vi "遥控器IP地址参数.vi"(10 "数组":u8[](array[numeric]), 11 "ID_VCU_MCU_1输入":u32=150013185 format="0x%x") -> (3 "Send":T1)   [LabVIEW 2016]
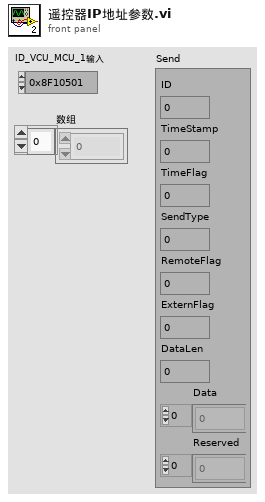
[diagram p1: front panel]
types:
  T1 = typedef "ControlCAN.lvlib/VCI_CAN_OBJ.ctl" = cluster{"ID":u32, "TimeStamp":u32, "TimeFlag":u8, "SendType":u8, "RemoteFlag":u8, "ExternFlag":u8, "DataLen":u8, "Data":u8[], "Reserved":u8[]}
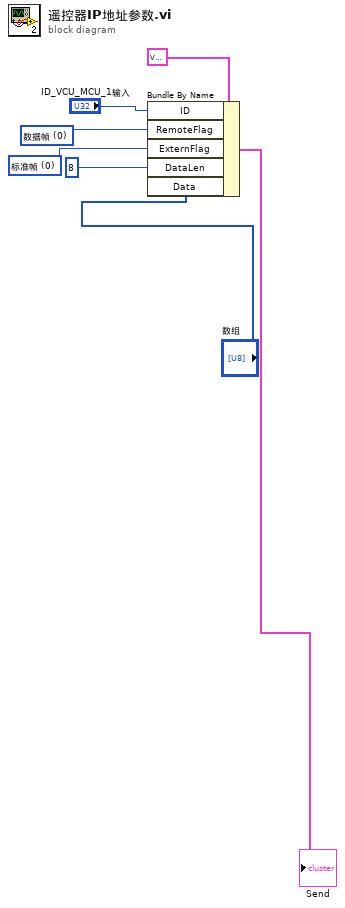
[diagram p0: block diagram]
diagram:
  w4 = u8 0 items=["标准帧", "扩展帧"] ("Format 2")
  w5 = u8 0 items=["数据帧", "远程帧"] ("Type 2")
  n1 = Bundle By Name(cluster=T1 {"ID"=0, "TimeStamp"=0, "TimeFlag"=0, "SendType"=0, "RemoteFlag"=0, "ExternFlag"=0, "DataLen"=0, "Data"=[], "Reserved"=[]} ("Send"), "ID"="ID_VCU_MCU_1输入", "RemoteFlag"=w5, "ExternFlag"=w4, "DataLen"=u8 8, "Data"="数组") -> (→"Send":T1)
